vi "BaseTemplate_SetModifiedClassAttributes.vi"(0 "reference in":refnum<class "BaseTemplate.lvclass">, 2 "Class attributes":T1, 3 "Only unlock data? (F)":bool, 4 "Unlock data if error? (T)":bool=TRUE, 5 "error in (no error)":errorcluster) -> (14 "reference out":refnum<class "BaseTemplate.lvclass">, 19 "error out":errorcluster)   [LabVIEW 2012, in "BaseTemplate.lvclass"]
doc: "This VI overwrites the class attributes associated with this class or subclass object reference and unlocks it for write access. If error in is set, the object is unlocked but its data will not be modified. If reference is wired, the class attributes of the class (or sub class) will be affected else the class attributes will default to the class.\n\nIn order to use this VI, you must first successfully lock the object's data using this class GetClassAttributesToModify VI."
uses:
  <resource>/Framework/Providers/Open_GDS/ClassProviders/Provider_EndevoGOOP300/Templates/BaseTemplate/BaseTemplate.lvclass
  <resource>/Framework/Providers/Open_GDS/ClassProviders/Provider_EndevoGOOP300/Templates/BaseTemplate/protected/ClassAttributes.ctl
  <resource>/Framework/Providers/Open_GDS/ClassProviders/Provider_EndevoGOOP300/Templates/BaseTemplate/BaseTemplate.lvclass/BaseTemplate.ctl
  <vilib>/addons/_goop3.llb/3GOOPStates.ctl
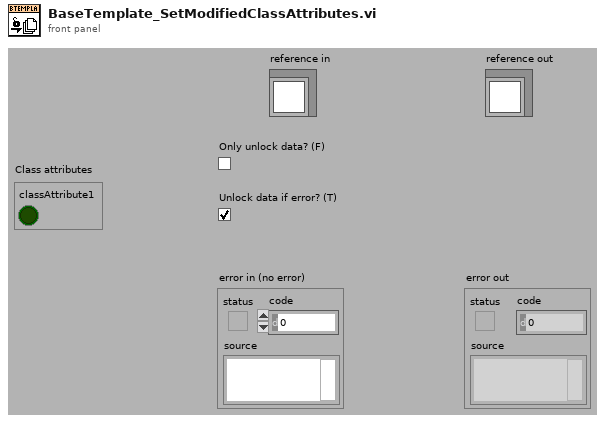
[diagram p1: front panel]
types:
  T1 = typedef "BaseTemplate.lvclass/ClassAttributes.ctl" = cluster{"classAttribute1":bool}
  T2 = typedef "BaseTemplate.lvclass/ObjectReference.ctl" = refnum<k1>
  T3 = typedef "3GOOPStates.ctl" = enum16{"Set", "Get", "New", "Delete", "Clear", "Test and get", "Unlock data", "Information", "Look up existing", "New or look up existing", "Test and get shared", "Get shared", "Set shared", "Unlock shared", "Find dynamic method", "Register dynamic method", "Preload dynamic method", "Probe", "Cast to more generic", "Cast to more specific"}
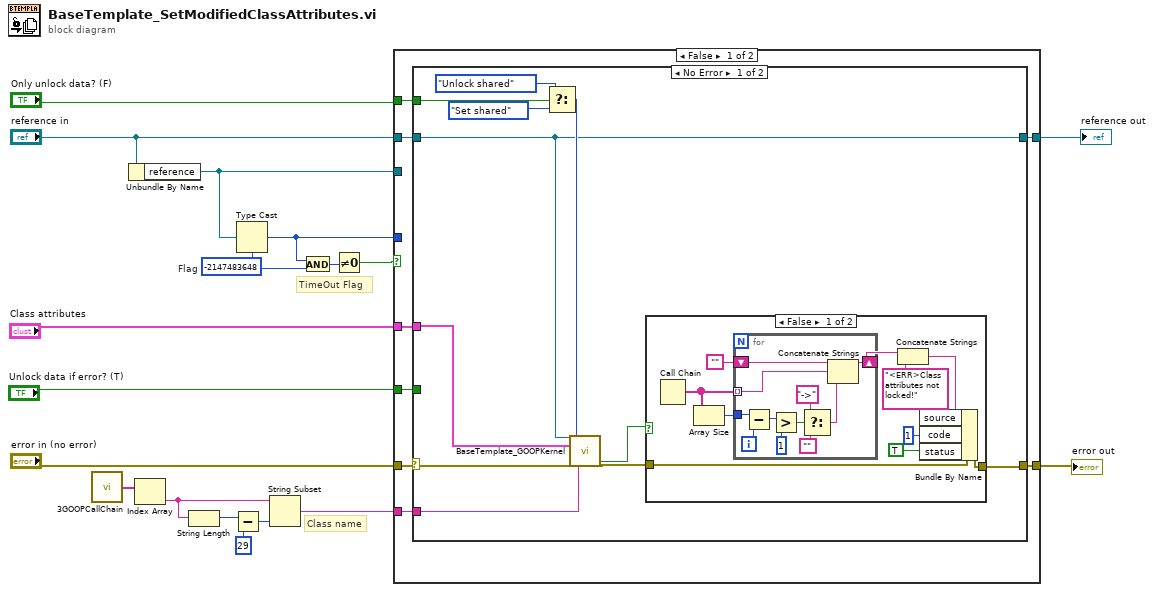
[diagram p0: block diagram]
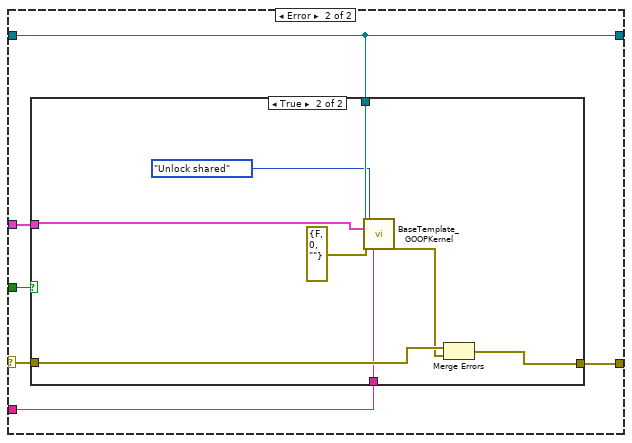
[diagram p3: hidden frame]
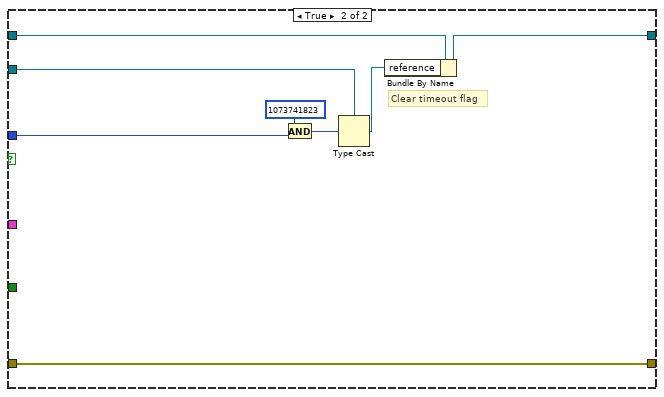
[diagram p5: hidden frame]
diagram:
  w10 = -2147483648  # Flag
  # "TimeOut Flag"
  # "Class name"
  n1 = call <vilib>:"3GOOPCallChain.vi"() -> ("call chain"=w15:string[])
  n2 = Unbundle By Name("reference in") -> ("reference"=w12:T2)
  n3 = Index Array(array=w15) -> (element=w18:string)  [unwired: 1 in]
  n4 = String Length(string=w18) -> (length=w14:i32)
  n5 = Subtract(x=w14, y=29) -> (x-y=w16:i32)
  n6 = Type Cast(type=w10, x=w12) -> (*(type *) &x=w11:i32)
  n7 = String Subset(string=w18, length (rest)=w16) -> (substring=w3:string)  [unwired: 1 in]
  n8 = And(x=w11, y=w10) -> (x .and. y?=w13:i32)
  n9 = Not Equal To 0?(x=w13) -> (x != 0?=w4:bool)
  n10 = case shown="False" w4 {
    tunnel: [w26 w78] -> w9
    tunnel: "Class attributes" -> [w25 _]
    tunnel: [w24 w77] -> w8
    tunnel: "Only unlock data? (F)" -> [w23 _]
    tunnel: "Unlock data if error? (T)" -> [w22 _]
    tunnel: "error in (no error)" -> [w21 w77]
    tunnel: "reference in" -> [w20 w79]
    tunnel: w12 -> [_ w76]
    tunnel: w11 -> [_ w75]
    tunnel: w3 -> [w19 _]
    frame False {
      n11 = case shown="No Error" w21 {
        selector: w21 -> [w37 w64]
        tunnel: [w32 w61] -> w26
        tunnel: w25 -> [w29 w63]
        tunnel: [w33 w62] -> w24
        tunnel: w20 -> [w32 w61]
        tunnel: w23 -> [w27 _]
        tunnel: w22 -> [_ w65]
        tunnel: w19 -> [w28 w60]
        frame No Error {
          n12 = Select(t=3GOOPStates."Unlock shared" ("Action"), s=w27, f=3GOOPStates."Set shared" ("Action")) -> (s? t:f=w34:T3)
          n13 = call <resource>:"BaseTemplate_GOOPKernel.vi"("Ref in"=w32, "Data shared in"=w29, "error in (no error)"=w37, "Action"=w34, "Class name"=w28) -> ("Data locked?"=w30:bool, "error out"=w31:errorcluster)  [unwired: 12 in, 9 out]
          n14 = case shown="False" w30 {
            tunnel: w31 -> [w42 w59]
            tunnel: [w43 w59] -> w33
            frame False {
              n15 = Call Chain() -> (call chain=w38:string[])
              n16 = Array Size(array=w38) -> (size(s)=w46:i32)
              n17 = for {
                shift-right: [w52] -> w45
                shift-left: "" -> [w54]
                tunnel: w38 -> [w53] mode=indexing
                tunnel: w46 -> [w58]
                i -> [w57]
                n18 = Subtract(x=w58, y=w57) -> (x-y=w56:i32)
                n19 = Greater?(x=w56, y=1) -> (0:w49:bool)
                n20 = Select(t="->", s=w49, f="") -> (s? t:f=w48:string)
                n21 = Concatenate Strings(w54, w53, w48) -> (w52:string)
              }
              n22 = Concatenate Strings(w45, "<ERR>Class attributes not locked!" ("Bundle Element")) -> (w41:string)
              n23 = Bundle By Name(cluster=w42, "source"=w41, "code"=1, "status"=TRUE) -> (w43:errorcluster)
            }
            frame True {
            }
          }
        }
        frame Error {
          n24 = case shown="True" w65 {
            tunnel: w64 -> [w66 w73]
            tunnel: [w66 w74] -> w62
            tunnel: w63 -> [_ w68]
            tunnel: w61 -> [_ w70]
            tunnel: w60 -> [_ w67]
            frame False {
            }
            frame True {
              n25 = call <resource>:"BaseTemplate_GOOPKernel.vi"("Ref in"=w70, "Data shared in"=w68, "error in (no error)"=errorcluster {"status"=FALSE, "code"=0, "source"=""}, "Action"=3GOOPStates."Unlock shared", "Class name"=w67) -> ("error out"=w71:errorcluster)  [unwired: 12 in, 10 out]
              n26 = Merge Errors(w73, w71) -> (w74:errorcluster)
            }
          }
        }
      }
    }
    frame True {
      # "Clear timeout flag"
      n27 = And(x=1073741823 ("x .and. y?"), y=w75) -> (x .and. y?=w81:i32)
      n28 = Type Cast(type=w76, x=w81) -> (*(type *) &x=w82:T2)
      n29 = Bundle By Name(cluster=w79, "reference"=w82) -> (w78:refnum<class "BaseTemplate.lvclass">)
    }
  }
  "error out" <- w8
  "reference out" <- w9
